vi "DC meter manual control GUI.vi"(11 "DC meter":T1) -> ()   [LabVIEW 2020]
doc: "GUI to manally controll the DC meter."
uses:
  Type definitions/DC meter.ctl
  Type definitions/DC meter type.ctl
  <vilib>/Utility/error.llb/Error Cluster From Error Code.vi
  <vilib>/ErrorRing/Error Ring.xnode
  external libraries/varilib/varilib.lvlib
panel:
  out "Waveform Graph":dbl[](graph)
  out "DC readings":dbl[](array[numeric])
  in  "No of readings":i32=1
  out "error out":errorcluster
  in  "stop":bool
  in  "read":bool
  out "gui_elements":refnum<vi>[](array[refnum])
  out "Status":string
  in  "initialize":bool
  in  "quit":bool
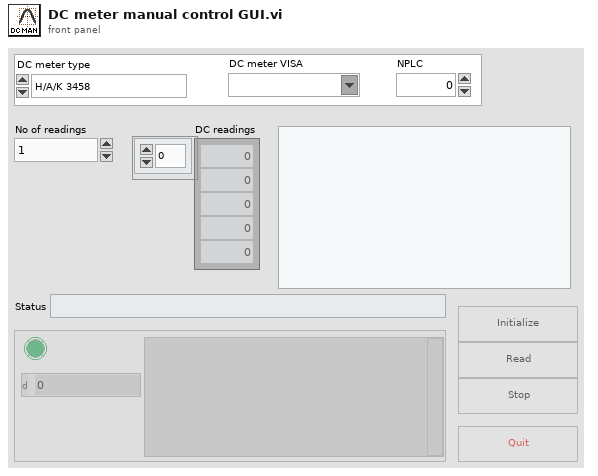
[diagram p1: front panel]
types:
  T1 = typedef "DC meter.ctl" = cluster{"DC meter type":T2, "DC meter VISA":refnum<visa-resource-name>, "NPLC":dbl, "status ref":refnum<vi>}
  T2 = typedef "DC meter type.ctl" = enum16{"H/A/K 3458", "Fluke 8508A", "dummy", "Keithley 2182"}
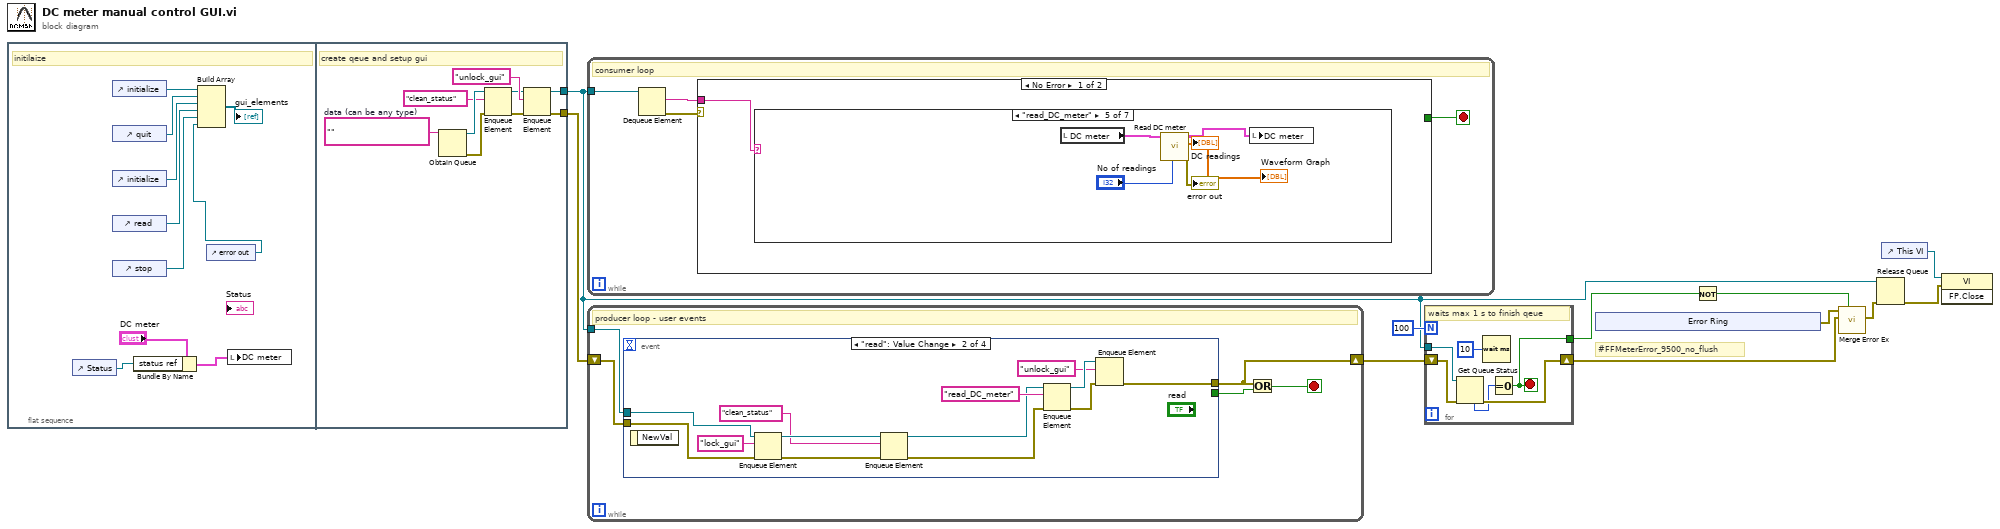
[diagram p0: block diagram]
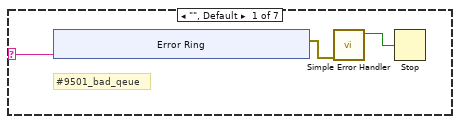
[diagram p2: hidden frame]
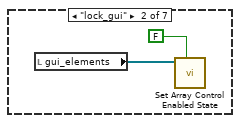
[diagram p3: hidden frame]
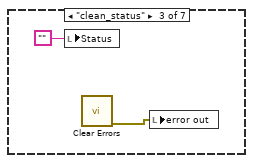
[diagram p4: hidden frame]
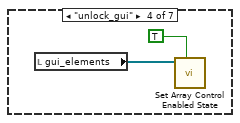
[diagram p5: hidden frame]
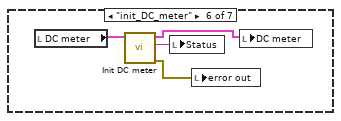
[diagram p6: hidden frame]
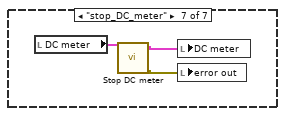
[diagram p7: hidden frame]
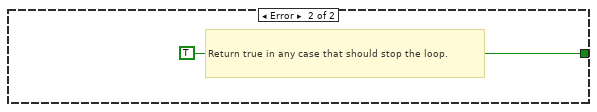
[diagram p8: hidden frame]
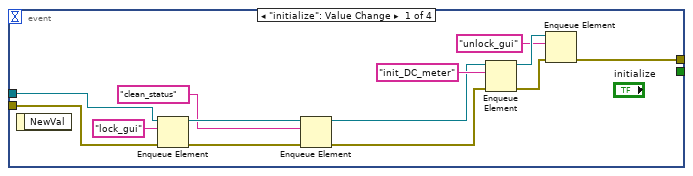
[diagram p9: hidden frame]
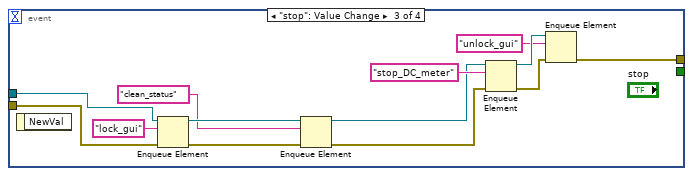
[diagram p10: hidden frame]
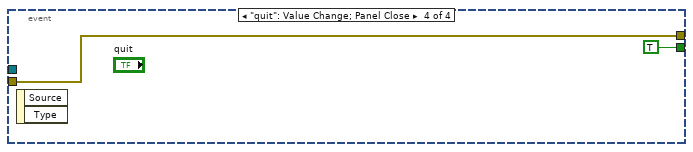
[diagram p11: hidden frame]
diagram:
  # "#FFMeterError_9500_no_flush"
  n1 = flat-sequence {
    tunnel: [w26] -> w4
    tunnel: [w24] -> w3
    frame #0 {
      # "initilaize"
      n2 = control-ref of="Status"() -> (w12:refnum<vi>)
      n3 = control-ref of="initialize"() -> (w21:refnum<vi>)
      n4 = control-ref of="quit"() -> (w20:refnum<vi>)
      n5 = control-ref of="initialize"() -> (w16:refnum<vi>)
      n6 = control-ref of="read"() -> (w17:refnum<vi>)
      n7 = control-ref of="stop"() -> (w18:refnum<vi>)
      n8 = Bundle By Name(cluster="DC meter", "status ref"=w12) -> (w13:T1)
      n9 = control-ref of="error out"() -> (w15:refnum<vi>)
      n10 = Build Array(w21, w20, w16, w17, w18, w15) -> (→"gui_elements":refnum<vi>[])
      n11 = local write "DC meter"(w13) -> ()
    }
    frame #1 {
      w25 = ""  # data (can be any type)
      # "create qeue and setup gui"
      n12 = Obtain Queue(element data type=w25) -> (queue out=w29:refnum<queue>, error out=w30:errorcluster)  [unwired: 4 in, 1 out]
      n13 = Enqueue Element(queue=w29, element="clean_status", error in (no error)=w30) -> (queue out=w22:refnum<queue>, error out=w23:errorcluster)  [unwired: 1 in, 1 out]
      n14 = Enqueue Element(queue=w22, element="unlock_gui", error in (no error)=w23) -> (queue out=w26:refnum<queue>, error out=w24:errorcluster)  [unwired: 1 in, 1 out]
    }
  }
  n15 = while {
    tunnel: w4 -> [w34]
    stop <- w31 stop-if-true
    # "consumer loop"
    n16 = Dequeue Element(queue=w34) -> (element=w32:string, error out=w33:errorcluster)  [unwired: 2 in, 2 out]
    n17 = case shown="No Error" w33 {
      tunnel: w32 -> [w35 _]
      tunnel: [_ TRUE] -> w31
      frame No Error {
        n18 = case shown="\"read_DC_meter\"" w35 {
          selector: w35 -> [w36 _ _ _ _ _ _]
          frame "", Default {
            # "#9501_bad_qeue"
            n19 = xnode "Error Ring"("parameter 0"=w36) -> ("error out"=w38:errorcluster)
            n20 = call <vilib>:"Simple Error Handler.vi"("error in (no error)"=w38) -> ("error?"=w37:bool)  [unwired: 4 in, 4 out]
            n21 = Stop(stop? (T)=w37) -> ()
          }
          frame "lock_gui" {
            n22 = local read "gui_elements"() -> (w47:refnum<vi>[])
            n23 = call "Set Array Control Enabled State.vi"("enabled (T)"=FALSE, "reference array in"=w47) -> ()  [unwired: 8 in, 2 out]
          }
          frame "clean_status" {
            n24 = local write "Status"("") -> ()
            n25 = call <vilib>:"Clear Errors.vi"() -> ("error out"=w48:errorcluster)  [unwired: 6 in, 1 out]
            n26 = local write "error out"(w48) -> ()
          }
          frame "unlock_gui" {
            n27 = local read "gui_elements"() -> (w51:refnum<vi>[])
            n28 = call "Set Array Control Enabled State.vi"("enabled (T)"=TRUE, "reference array in"=w51) -> ()  [unwired: 8 in, 2 out]
          }
          frame "read_DC_meter" {
            n29 = local read "DC meter"() -> (w56:T1)
            n30 = call "Read DC meter.vi"("No of readings"="No of readings", "DC meter"=w56) -> ("error out"=→"error out":errorcluster, "DC readings"=→"DC readings" →"Waveform Graph":dbl[], "DC meter out"=w55:T1)  [unwired: 7 in]
            n31 = local write "DC meter"(w55) -> ()
          }
          frame "init_DC_meter" {
            n32 = local read "DC meter"() -> (w59:T1)
            n33 = call "Init DC meter.vi"("DC meter"=w59) -> ("error out"=w60:errorcluster, "Init status"=w57:string, "DC meter out"=w58:T1)  [unwired: 8 in]
            n34 = local write "Status"(w57) -> ()
            n35 = local write "error out"(w60) -> ()
            n36 = local write "DC meter"(w58) -> ()
          }
          frame "stop_DC_meter" {
            n37 = local read "DC meter"() -> (w61:T1)
            n38 = call "Stop DC meter.vi"("DC meter"=w61) -> ("error out"=w63:errorcluster, "DC meter out"=w62:T1)  [unwired: 9 in]
            n39 = local write "DC meter"(w62) -> ()
            n40 = local write "error out"(w63) -> ()
          }
        }
      }
      frame Error {
        # "Return true in any case that should stop the loop."
      }
    }
  }
  n41 = while {
    shift-right: [w65] -> w7
    shift-left: w3 -> [w68]
    tunnel: w4 -> [w69]
    stop <- w66 stop-if-true
    # "producer loop - user events"
    n42 = event shown="[1] \"read\": Value Change" {
      selector: _ -> [_ _ _ _]
      dyn-events: _ -> [_ _ _ _]
      timeout: _ -> [_ _ _ _]
      tunnel: w69 -> [w76 w89 w102 _]
      tunnel: w68 -> [w77 w90 w103 w110]
      tunnel: [w80 w93 w106 w110] -> w65
      tunnel: [_ _ _ TRUE ("cancel")] -> w67
      event "initialize": Value Change {
        n43 = event-data() -> ()  [unwired: 1 in, 1 out]
        n44 = Enqueue Element(queue=w76, element="lock_gui", error in (no error)=w77) -> (queue out=w73:refnum<queue>, error out=w74:errorcluster)  [unwired: 1 in, 1 out]
        n45 = Enqueue Element(queue=w73, element="clean_status", error in (no error)=w74) -> (queue out=w71:refnum<queue>, error out=w70:errorcluster)  [unwired: 1 in, 1 out]
        n46 = Enqueue Element(queue=w71, element="init_DC_meter", error in (no error)=w70) -> (queue out=w79:refnum<queue>, error out=w81:errorcluster)  [unwired: 1 in, 1 out]
        n47 = Enqueue Element(queue=w79, element="unlock_gui", error in (no error)=w81) -> (error out=w80:errorcluster)  [unwired: 1 in, 2 out]
      }
      event "read": Value Change {
        n48 = event-data() -> ()  [unwired: 1 in, 1 out]
        n49 = Enqueue Element(queue=w89, element="lock_gui", error in (no error)=w90) -> (queue out=w86:refnum<queue>, error out=w87:errorcluster)  [unwired: 1 in, 1 out]
        n50 = Enqueue Element(queue=w86, element="clean_status", error in (no error)=w87) -> (queue out=w84:refnum<queue>, error out=w83:errorcluster)  [unwired: 1 in, 1 out]
        n51 = Enqueue Element(queue=w84, element="read_DC_meter", error in (no error)=w83) -> (queue out=w92:refnum<queue>, error out=w94:errorcluster)  [unwired: 1 in, 1 out]
        n52 = Enqueue Element(queue=w92, element="unlock_gui", error in (no error)=w94) -> (error out=w93:errorcluster)  [unwired: 1 in, 2 out]
      }
      event "stop": Value Change {
        n53 = event-data() -> ()  [unwired: 1 in, 1 out]
        n54 = Enqueue Element(queue=w102, element="lock_gui", error in (no error)=w103) -> (queue out=w99:refnum<queue>, error out=w100:errorcluster)  [unwired: 1 in, 1 out]
        n55 = Enqueue Element(queue=w99, element="clean_status", error in (no error)=w100) -> (queue out=w97:refnum<queue>, error out=w96:errorcluster)  [unwired: 1 in, 1 out]
        n56 = Enqueue Element(queue=w97, element="stop_DC_meter", error in (no error)=w96) -> (queue out=w105:refnum<queue>, error out=w107:errorcluster)  [unwired: 1 in, 1 out]
        n57 = Enqueue Element(queue=w105, element="unlock_gui", error in (no error)=w107) -> (error out=w106:errorcluster)  [unwired: 1 in, 2 out]
      }
      event "quit": Value Change; Panel Close {
        n58 = event-data() -> ()  [unwired: 1 in, 2 out]
      }
    }
    n59 = Or(x=w65, y=w67) -> (x .or. y?=w66:bool)
  }
  n60 = for {
    N: 100 -> [_]
    tunnel: w4 -> [w116]
    shift-right: [w114] -> w8
    shift-left: w7 -> [w115]
    tunnel: [w111] -> w5
    stop <- w111 stop-if-true
    # "waits max 1 s to finish qeue"
    n61 = Get Queue Status(queue=w116, error in (no error)=w115) -> (error out=w114:errorcluster, # elements in queue=w112:i32)  [unwired: 1 in, 6 out]
    n62 = Wait (ms)(milliseconds to wait=u32 10) -> ()  [unwired: 1 out]
    n63 = Equal To 0?(x=w112) -> (x = 0?=w111:bool)
  }
  n64 = xnode "Error Ring"() -> ("error out"=w9:errorcluster)
  n65 = Not(x=w5) -> (.not. x?=w10:bool)
  n66 = call "Merge Error Ex.vi"("Is error? (False)"=w10, "main error in (no error)"=w8, "second error in"=w9) -> ("error out"=w6:errorcluster)  [unwired: 8 in]
  n67 = Release Queue(queue=w4, error in (no error)=w6) -> (error out=w2:errorcluster)  [unwired: 1 in, 2 out]
  n68 = control-ref of="This VI"() -> (w1:refnum<vi>)
  n69 = invoke class="VI" method="FP.Close"(reference=w1, error in=w2) -> ()  [unwired: 1 in, 3 out]
